vi "TCP Write (Synchronous) - Send Message and Test Response.vi"(7 "Expected Response":string, 8 "error in":errorcluster, 9 "Timeout (ms)":i32, 10 "Data to Write":string, 11 "TCP Network Connecion In":refnum<k5>) -> (0 "error out":errorcluster, 1 "Actual Response":string, 2 "Valid Response":bool, 3 "TCP Network Connecion Out":refnum<k5>)   [LabVIEW 2017, in "Communications Library.lvlib"]
doc: "Synchronous write to TCP connection.\n\nSends a message through a TCP connection ands wait for the response message."
uses:
  Communications Library.lvlib
  Error 5102 - DTACQ unit replied with an error--const.vi
  Debug - TCP - Write to Log File.vi
  Debug - TCP - Create Descriptive String.vi
  <vilib>/Utility/error.llb/Error Cluster From Error Code.vi
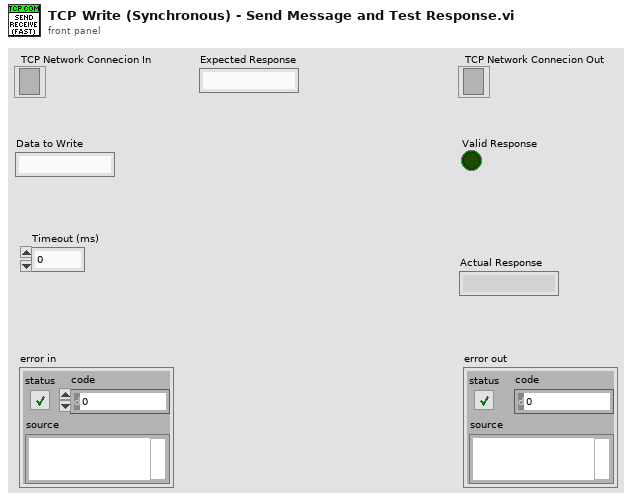
[diagram p1: front panel]
types:
  T1 = enum16{"Standard", "Buffered", "CRLF", "Immediate"}
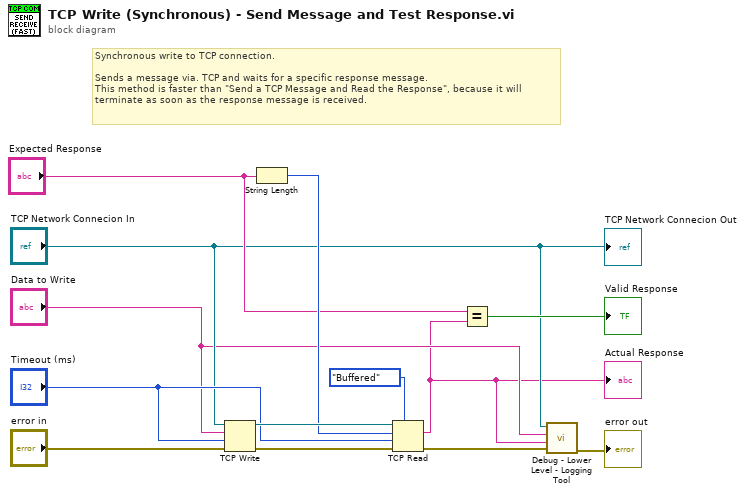
[diagram p0: block diagram]
diagram:
  # "Synchronous write to TCP connection.\n\nSends a message via. TCP and waits for a specific response message.\nThis method is faster than \"Send a TCP Message and Read the Response\", because it will\nterminate as soon as the response message is received."
  n1 = TCP Write(connection ID="TCP Network Connecion In", data in="Data to Write", error in (no error)="error in", 9:"Timeout (ms)") -> (connection ID out=w11:refnum<k5>, error out=w12:errorcluster)  [unwired: 1 out]
  n2 = String Length(string="Expected Response") -> (length=w9:i32)
  n3 = TCP Read(connection ID=w11, bytes to read=w9, error in (no error)=w12, 7:T1."Buffered" ("mode (standard)"), 9:"Timeout (ms)") -> (data out=w1:string, error out=w5:errorcluster)  [unwired: 1 out]
  "Actual Response" <- w1
  n4 = Equal?(x="Expected Response", y=w1) -> (x = y?=→"Valid Response":bool)
  n5 = call "Debug - Lower Level - Logging Tool.vi"("Error In"=w5, "Data Received"=w1, "Data Sent"="Data to Write", "TCP Network Connecion In"="TCP Network Connecion In") -> ("Error Out"=→"error out":errorcluster)  [unwired: 6 in, 1 out]
  "TCP Network Connecion Out" <- "TCP Network Connecion In"
